vi "From Variant.vi"(8 "Error In":errorcluster, 10 "Variant":variant, 11 "TD Bool In":refnum<class "Bool.lvclass">) -> (0 "Error Out":errorcluster, 3 "TD Bool Out":refnum<class "Bool.lvclass">)   [LabVIEW 2017, in "Tree API.lvlib" / "Bool.lvclass"]
doc: "Dynamic dispatch interface for conversion of variant LV data to Tree Data classes."
uses:
  Bool.lvclass
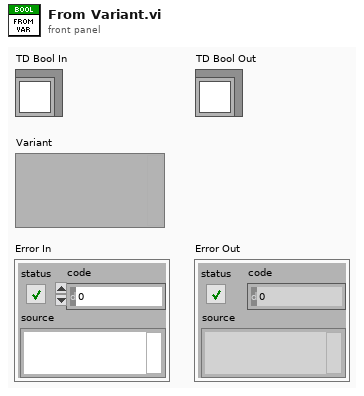
[diagram p1: front panel]
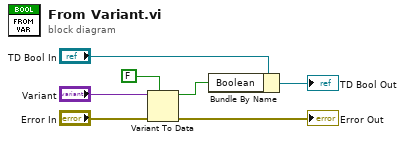
[diagram p0: block diagram]
diagram:
  n1 = Variant To Data(error in="Error In", type=FALSE ("Boolean"), Variant="Variant") -> (data=w2:bool, error out=→"Error Out":errorcluster)
  n2 = Bundle By Name(cluster="TD Bool In", "Boolean"=w2) -> (→"TD Bool Out":refnum<class "Bool.lvclass">)
